vi "BRig_RT__Case_Exp__State_ENL.vi"(0 "input_dataCurrent":u16[](array[numeric]), 1 "input_dataTrial":u16[][](array[numeric]), 5 "input_arrTrig":bool[](array[boolean]), 6 "input_state":T1, 8 "I_lick":bool) -> (7 "output_l2_laserOn":bool, 9 "output_l2_laserEvent":bool, 11 "output_l1_laserOn":bool, 12 "output_state":T1, 13 "output_l1_laserEvent":bool, 14 "output_dataCurrent":u16[](array[numeric]), 15 "output_dataTrial":u16[][](array[numeric]))   [LabVIEW 2014]
uses:
  myRIO_BRig_RT__Case_Exp_stateList.ctl
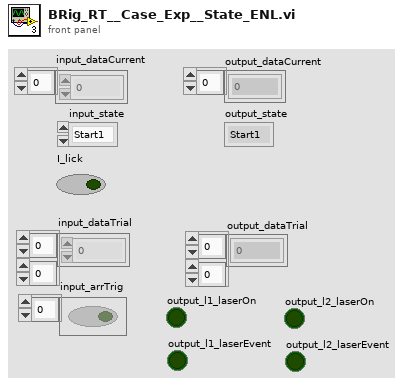
[diagram p1: front panel]
types:
  T1 = typedef "myRIO_BRig_RT__Case_Exp_stateList.ctl" = enum16{"Start1", "Start2", "Start3", "saveSettings1", "saveSettings2", "saveSettings3", "saveSettings4", "saveSettings_LC_ENL_l1", "saveSettings_LC_ENL_l2", "saveSettings_LC_Cue_l1", "saveSettings_LC_Cue_l2", "saveSettings6_LC_l1_Other", "SaveSettings6_LC_l2_Other", "setSettings_Audio", "setSettings_Laser", "initBlock_pre", "initBlock", "initBlock2", "initBlock_post", "initTrial_pre", "initTrial", "initTrial2", "initTrial3", "initTrial4", "initTrial_LC_ENL1", "initTrial_LC_Cue1", "initTrial_LC_Cue1_2", "initTrial_LC_Sel", "initTrial_post", "ENL1_pre", "ENL1", "ENL1_post", "ENL1Penalty_pre", "ENL1Penalty", "ENL2_pre", "ENL2", "ENL2Penalty_pre", "ENL2Penalty", "Cue1_pre", "Cue1", "Cue1_post", "Cue1Penalty_pre", "Cue1Penalty", "Cue2_pre", "Cue2", "Cue2Penalty_pre", "Cue2Penalty", "Selection_pre", "Selection", "Select_post", "SelectReward_pre", "SelectReward", "SelectRewardPost_pre", "SelectRewardPost", "SelectWrong_pre", "SelectWrong", "SelectWrong_post", "SelectTimeout_pre", "SelectTimeout", "SelectTimeout_post", "endTrial_pre", "endTrial1", "endTrial2", "endTrial3", "endTrial_post", "endBlock_pre", "endBlock", "endBlock_post", "endExp", "commConnect", "commUpload_pre", "commUpload_dataBlock", "commUpload_dataCurrent", "commUpload_dataExp", "commUpload_dataLC", "commUpload_dataTrial", "commUpload_post", "saveData_pre", "saveData_dataBlock", "saveData_dataCurrent", "saveData_dataExp", "saveData_dataLC", "saveData_dataTrial", "saveData_post", "empty_endBlock1", "empty_endBlock2", "empty_endTrial1", "empty_endTrial2", "empty_endTrial3", "empty_endTrial4", "empty_endTrial5", "dummyState", "dummyState_endBlock", "FreeReward_pre", "FreeReward", "FreeRewardPost_pre", "FreeRewardPost"}
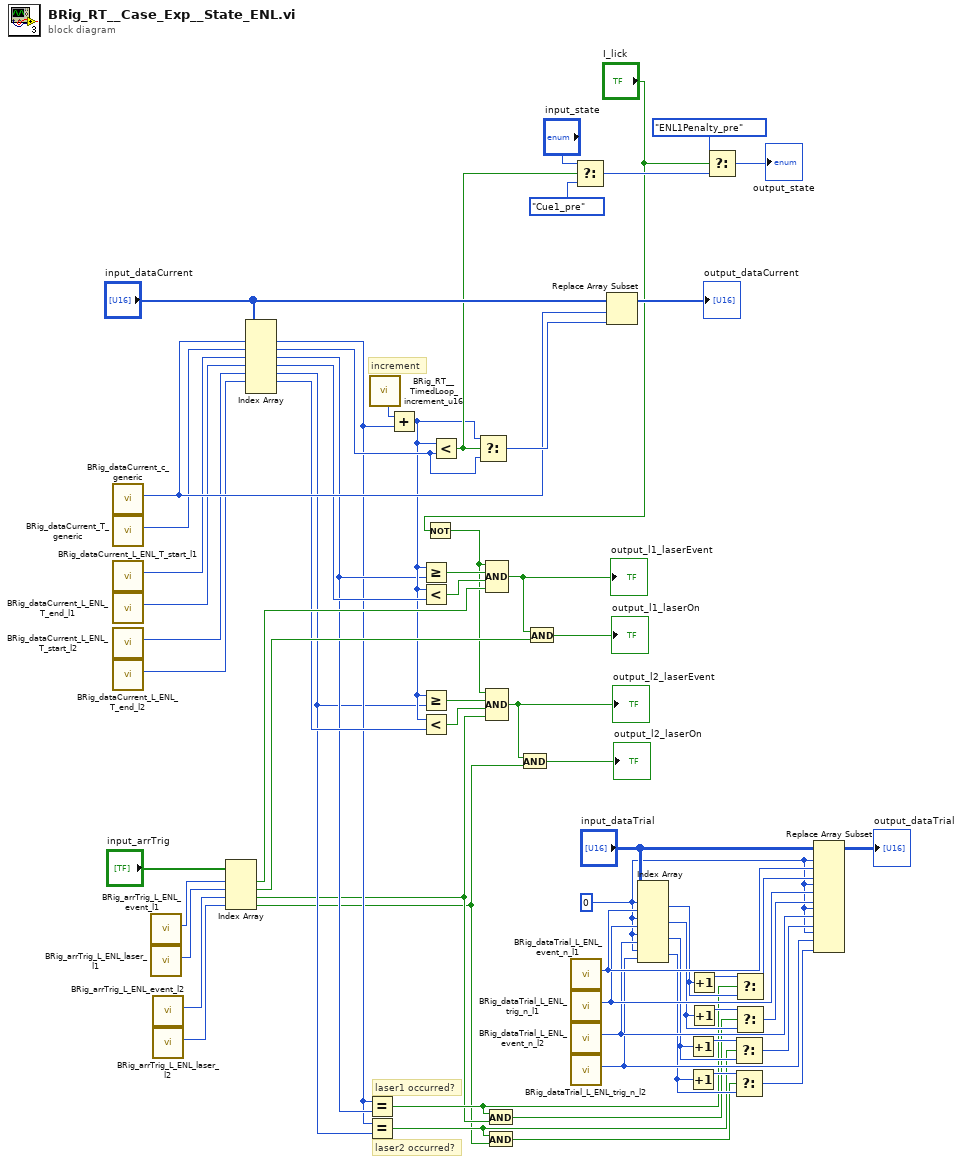
[diagram p0: block diagram]
diagram:
  w1 = 0
  # "laser2 occurred?"
  # "laser1 occurred?"
  # "increment"
  n1 = call "BRig_dataCurrent_c_generic.vi"() -> ("output_count_generic"=w46:i32)  [unwired: 11 in]
  n2 = call "BRig_dataCurrent_T_generic.vi"() -> ("output_T_generic"=w45:i32)  [unwired: 11 in]
  n3 = call "BRig_dataCurrent_L_ENL_T_start_l1.vi"() -> ("output_L_ENL_T_start_l1"=w43:i32)  [unwired: 11 in]
  n4 = call "BRig_dataCurrent_L_ENL_T_end_l1.vi"() -> ("output_L_ENL_T_end_l1"=w42:i32)  [unwired: 11 in]
  n5 = call "BRig_dataCurrent_L_ENL_T_start_l2.vi"() -> ("output_laser2_tENL1_start"=w41:i32)  [unwired: 11 in]
  n6 = call "BRig_dataCurrent_L_ENL_T_end_l2.vi"() -> ("output_L_ENL_T_end_l2"=w40:i32)  [unwired: 11 in]
  n7 = call "BRig_arrTrig_L_ENL_event_l1.vi"() -> ("output_L_ENL_event_l1"=w32:i32)  [unwired: 11 in]
  n8 = call "BRig_arrTrig_L_ENL_laser_l1.vi"() -> ("output_L_ENL_laserTrig_l1"=w31:i32)  [unwired: 11 in]
  n9 = call "BRig_arrTrig_L_ENL_event_l2.vi"() -> ("output_L_ENL_event_l2"=w30:i32)  [unwired: 11 in]
  n10 = call "BRig_arrTrig_L_ENL_laser_l2.vi"() -> ("output_L_ENL_laserTrig_l2"=w29:i32)  [unwired: 11 in]
  n11 = Index Array(array="input_arrTrig", index #1=w32, index #2=w31, index #3=w30, index #4=w29) -> (element #1=w37:bool, element #2=w36:bool, element #3=w10:bool, element #4=w9:bool)
  n12 = Index Array(array="input_dataCurrent", index #1=w46, index #2=w45, index #3=w43, index #4=w42, index #5=w41, index #6=w40) -> (element #1=w27:u16, element #2=w44:u16, element #3=w28:u16, element #4=w38:u16, element #5=w26:u16, element #6=w33:u16)  [unwired: 1 in, 1 out]
  n13 = Equal?(x=w27, y=w28) -> (x = y?=w12:bool)
  n14 = Equal?(x=w27, y=w26) -> (x = y?=w11:bool)
  n15 = call "BRig_RT__TimedLoop_increment_u16.vi"() -> ("output_increment__u16"=w60:u16)  [unwired: 11 in]
  n16 = Add(x=w60, y=w27) -> (x+y=w34:u16)
  n17 = Greater Or Equal?(x=w34, y=w28) -> (x >= y?=w58:bool)
  n18 = Less?(x=w34, y=w38) -> (x < y?=w59:bool)
  n19 = Greater Or Equal?(x=w34, y=w26) -> (x >= y?=w50:bool)
  n20 = Less?(x=w34, y=w33) -> (x < y?=w49:bool)
  n21 = Not(x="I_lick") -> (.not. x?=w35:bool)
  n22 = Less?(x=w34, y=w44) -> (x < y?=w62:bool)
  n23 = Select(t=w34, s=w62, f=w44) -> (s? t:f=w63:u16)
  n24 = Compound Arithmetic op=AND(w35, w58, w59, w37) -> (w52:bool)
  "output_l1_laserEvent" <- w52
  n25 = Compound Arithmetic op=AND(w35, w50, w49, w10) -> (w48:bool)
  "output_l2_laserEvent" <- w48
  n26 = And(x=w12, y=w10) -> (x .and. y?=w8:bool)
  n27 = And(x=w11, y=w9) -> (x .and. y?=w7:bool)
  n28 = And(x=w48, y=w9) -> (x .and. y?=→"output_l2_laserOn":bool)
  n29 = And(x=w52, y=w36) -> (x .and. y?=→"output_l1_laserOn":bool)
  n30 = call "BRig_dataTrial_L_ENL_event_n_l1.vi"() -> ("output_L_ENL_event_n_l1"=w24:i32)  [unwired: 11 in]
  n31 = call "BRig_dataTrial_L_ENL_trig_n_l1.vi"() -> ("output_L_ENL_trig_n_l1"=w23:i32)  [unwired: 11 in]
  n32 = call "BRig_dataTrial_L_ENL_event_n_l2.vi"() -> ("output_L_ENL_event_n_l2"=w22:i32)  [unwired: 11 in]
  n33 = call "BRig_dataTrial_L_ENL_trig_n_l2.vi"() -> ("output_L_ENL_trig_n_l2"=w21:i32)  [unwired: 11 in]
  n34 = Select(t="input_state", s=w62, f=myRIO_BRig_RT__Case_Exp_stateList."Cue1_pre" ("Enum")) -> (s? t:f=w61:T1)
  n35 = Replace Array Subset(array="input_dataCurrent", new element=w63, index=w46) -> (→"output_dataCurrent":u16[])
  n36 = Index Array(array="input_dataTrial", index (row) #1=w1, index (col) #1=w24, index (row) #2=w1, index (col) #2=w23, index (row) #3=w1, index (col) #3=w22, index (row) #4=w1, index (col) #4=w21) -> (element #1=w19:u16, element #2=w15:u16, element #3=w14:u16, element #4=w13:u16)
  n37 = Increment(x=w14) -> (x+1=w17:u16)
  n38 = Increment(x=w13) -> (x+1=w16:u16)
  n39 = Increment(x=w19) -> (x+1=w20:u16)
  n40 = Increment(x=w15) -> (x+1=w18:u16)
  n41 = Select(t=myRIO_BRig_RT__Case_Exp_stateList."ENL1Penalty_pre" ("Enum"), s="I_lick", f=w61) -> (s? t:f=→"output_state":T1)
  n42 = Select(t=w17, s=w11, f=w14) -> (s? t:f=w4:u16)
  n43 = Select(t=w16, s=w7, f=w13) -> (s? t:f=w3:u16)
  n44 = Select(t=w20, s=w12, f=w19) -> (s? t:f=w6:u16)
  n45 = Select(t=w18, s=w8, f=w15) -> (s? t:f=w5:u16)
  n46 = Replace Array Subset(array="input_dataTrial", new element #1=w6, index (row) #1=w1, index (col) #1=w24, new element #2=w5, index (row) #2=w1, index (col) #2=w23, new element #3=w4, index (row) #3=w1, index (col) #3=w22, new element #4=w3, index (row) #4=w1, index (col) #4=w21) -> (→"output_dataTrial":u16[][])
